vi "Delete from Object.vi"(6 "$Path or Item Name":string, 7 "error in (no error)":errorcluster, 9 "Offset":i32 caption="Object Offset", 10 "JSON":string="{}") -> (0 "error out":errorcluster, 1 "<JSON>":string caption="<JSON>Deleted", 2 "Found and Deleted":bool, 3 "<JSON>":string caption="<JSON>With Item Deleted")   [LabVIEW 2017, in "JSONtext.lvlib"]
doc: "This function is DEPRECATED: please use \"Delete.vi\" instead.\n\nDeletes JSON item at the JSON Path specified. Only accepts paths that specify a unique Object item (no Arrays or multi-item lists), and thus only deletes one item. Use \"Delete.vi\" to delete multiple items."
uses:
  JSONtext.lvlib
  Parsing/Parsing State.ctl
  support/Quote and Escape JSON string.vi
  Parsing/Advance past whitespace.vi
  support/quote and escape json string 2.vi
  Parsing/Parse Full Path or Item Name.vi
  Parsing/Path Notation End Name.vi
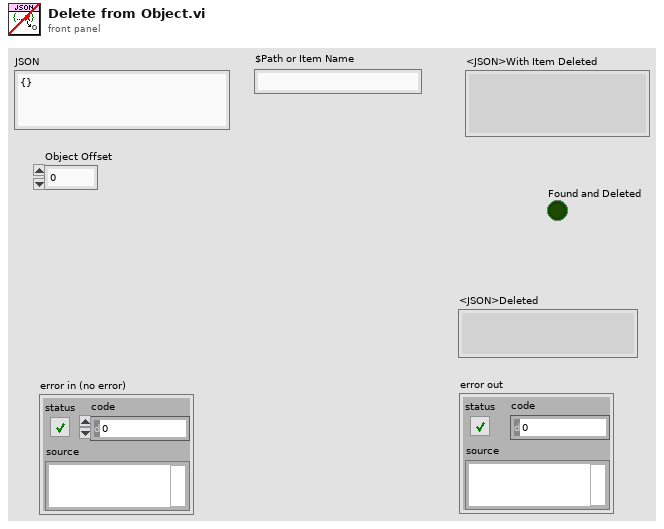
[diagram p1: front panel]
types:
  T1 = typedef "JSONtext.lvlib/Parsing State.ctl" = enum16{"Parser Error", "Object", "Array", "String", "Number/Other", "Leading Whitespace", "Object end", "Array end", "Value end"}
  T2 = typedef "JSONtext.lvlib/Found Items.ctl" = cluster{"Item offset":i32, "Offset past Item":i32, "Name offset":i32, "Offset past Name":i32, "Found":bool, "Item Type":T1, "Item Index":i32}
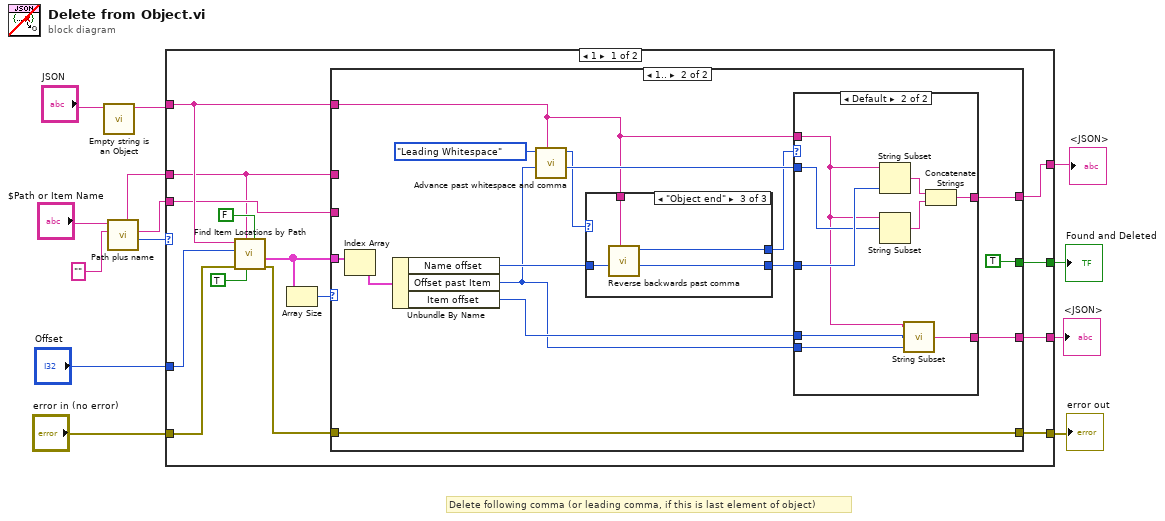
[diagram p0: block diagram]
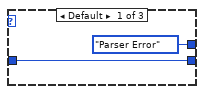
[diagram p3: hidden frame]
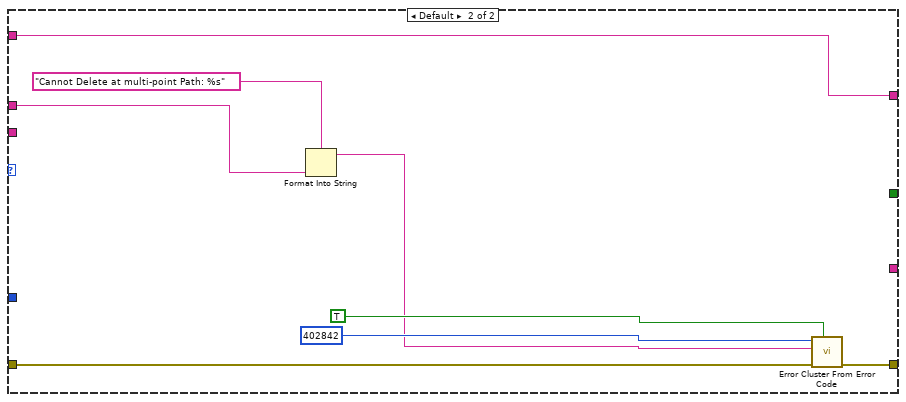
[diagram p6: hidden frame]
diagram:
  # "Delete following comma (or leading comma, if this is last element of object)"
  n1 = call "Empty string is an Object.vi"("JSON Input"="JSON") -> ("<JSON>Object"=w7:string)  [unwired: 10 in]
  n2 = call "Path plus name.vi"("Item Name"="", "Object (or Item) Path"="$Path or Item Name") -> ("Number of Paths"=w1:i32, "<JSON>End Name"=w2:string, "Relative Path or JSON-format name"=w3:string)  [unwired: 7 in]
  n3 = case shown="1" w1 {
    tunnel: [w27 w64] -> w13
    tunnel: w7 -> [w26 w64]
    tunnel: "Offset" -> [w25 _]
    tunnel: [w23 _] -> w11
    tunnel: "error in (no error)" -> [w22 w65]
    tunnel: [w15 w68] -> w9
    tunnel: w2 -> [w20 _]
    tunnel: w3 -> [w17 w63]
    tunnel: [w14 _] -> w6
    frame 1 {
      n4 = call "Find Item Locations by Path.vi"("Insertion point if not found"=FALSE, "Only return first found"=TRUE, "Path"=w17, "error in (no error)"=w22, "Offset"=w25, "JSON"=w26) -> ("error out"=w16:errorcluster, "Items"=w19:T2[])  [unwired: 4 in]
      n5 = Array Size(array=w19) -> (size(s)=w18:i32)
      n6 = case shown="1.." w18 {
        tunnel: [w29 w39] -> w27
        tunnel: w26 -> [w29 w36]
        tunnel: w19 -> [_ w44]
        tunnel: [_ TRUE] -> w23
        tunnel: w20 -> [_ _]
        tunnel: w16 -> [w28 w43]
        tunnel: w17 -> [_ _]
        tunnel: [w28 w43] -> w15
        tunnel: [_ w30] -> w14
        frame 0, Default {
        }
        frame 1.. {
          n7 = Index Array(array=w44) -> (element=w41:T2)  [unwired: 1 in]
          n8 = Unbundle By Name(w41) -> ("Name offset"=w38:i32, "Offset past Item"=w31:i32, "Item offset"=w32:i32)
          n9 = call "Advance past whitespace and comma.vi"("JSON"=w36, "Offset"=w31, "State in"=Parsing_State."Leading Whitespace") -> ("Offset past match"=w40:i32, "State"=w35:T1)  [unwired: 7 in]
          n10 = case shown="\"Object end\"" w35 {
            selector: w35 -> [_ w47 _]
            tunnel: w38 -> [w46 w48 w52]
            tunnel: [w46 w48 w51] -> w37
            tunnel: w36 -> [_ _ w50]
            tunnel: [Parsing_State."Parser Error" ("Parser State") w47 w49] -> w34
            frame Default {
            }
            frame "Object".."Number/Other" {
            }
            frame "Object end" {
              n11 = call "Reverse backwards past comma.vi"("JSON"=w50, "Offset"=w52) -> ("Offset of first non-whitespace"=w51:i32, "Parser State"=w49:T1)  [unwired: 8 in]
            }
          }
          n12 = case shown="Default" w34 {
            tunnel: w36 -> [w53 w57]
            tunnel: w37 -> [_ w62]
            tunnel: w40 -> [_ w61]
            tunnel: [w53 w58] -> w39
            tunnel: w32 -> [_ w56]
            tunnel: w31 -> [_ w55]
            tunnel: [_ w54] -> w30
            frame "Parser Error" {
            }
            frame Default {
              n13 = String Subset(string=w57, length (rest)=w62) -> (substring=w60:string)  [unwired: 1 in]
              n14 = String Subset(string=w57, offset (0)=w61) -> (substring=w59:string)  [unwired: 1 in]
              n15 = call "String Subset.vi"("Offset past End"=w55, "Start offset"=w56, "JSON"=w57) -> ("substring"=w54:string)  [unwired: 2 in]
              n16 = Concatenate Strings(w60, w59) -> (w58:string)
            }
          }
        }
      }
    }
    frame Default {
      n17 = Format Into String(format string="Cannot Delete at multi-point Path: %s", w63) -> (resulting string=w66:string)  [unwired: 2 in, 1 out]
      n18 = call <vilib>:"Error Cluster From Error Code.vi"("show call chain? (False)"=TRUE, "error in (no error)"=w65, "error message (\"\")"=w66, "error code (0)"=402842) -> ("error out"=w68:errorcluster)  [unwired: 5 in]
    }
  }
  "Found and Deleted" <- w11
  "<JSON>" <- w13
  "error out" <- w9
  "<JSON>" <- w6
